vi "loadCal.vi"(8 "error in (no error)":errorcluster, 9 "Wavelength Range (nm)":refnum<vi>, 10 "Center WL (nm)":refnum<vi>, 11 "Type of Measurement":u16(ring)=1 items=["Reflection", "Transmission"]) -> (0 "error out":errorcluster, 2 "valid?":bool)   [LabVIEW 2024]
uses:
  Program Files (x86)/Luna Technologies/OVA 5000 v5.14.2/data/OVA32.dll
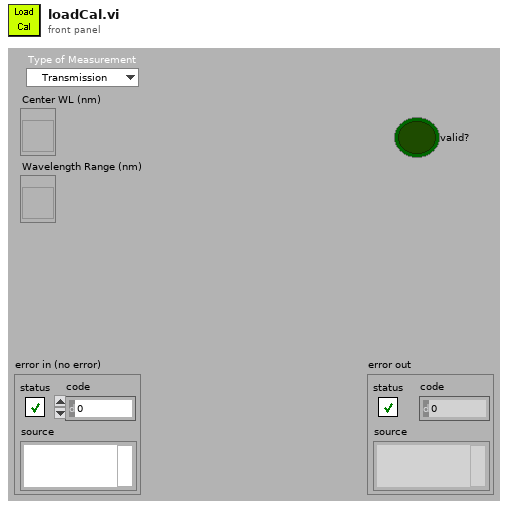
[diagram p1: front panel]
types:
  T1 = cluster{"calStartWL":dbl, "avgs":u32, "timeLength":dbl, "deciFactor":u32, "minStartWL":dbl, "rangeArray":dbl[], "minAvgs":u32, "maxAvgs":u32, "measType":u8, "timeStamp":string, "dutLength":dbl}
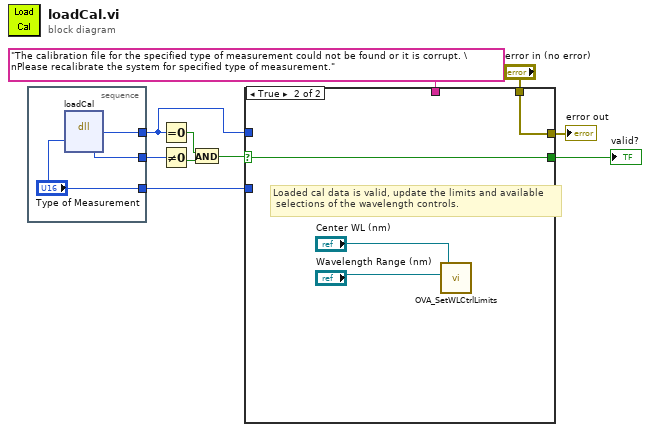
[diagram p0: block diagram]
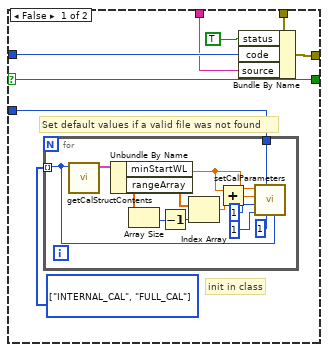
[diagram p2: hidden frame]
diagram:
  n1 = stacked-sequence {
    tunnel: [w13] -> w1
    tunnel: [w12] -> w7
    tunnel: ["Type of Measurement"] -> w6
    frame #0 {
      n2 = dll-call lib="C:/Program Files (x86)/Luna Technologies/OVA 5000 v5.14.2/data/OVA32.dll" fn="loadCal" label="loadCal()"("measType"="Type of Measurement") -> (w13:i32, "valid?"=w12:u8)  [unwired: 5 in, 2 out]
    }
  }
  n3 = Equal To 0?(x=w1) -> (x = 0?=w4:bool)
  n4 = Not Equal To 0?(x=w7) -> (x != 0?=w2:bool)
  n5 = And(x=w4, y=w2) -> (x .and. y?=w3:bool)
  n6 = case shown="True" w3 {
    selector: w3 -> [w14 w34]
    tunnel: "error in (no error)" -> [w21 w37]
    tunnel: [w20 w37] -> w8
    tunnel: w1 -> [w19 _]
    tunnel: "The calibration file for the specified type of measurement could not be found or it is corrupt. \nPlease recalibrate the system for specified type of measurement." -> [w17 _]
    tunnel: w6 -> [w16 _]
    tunnel: [w14 w34] -> w5
    frame False {
      w15 = enum16{"INTERNAL_CAL", "FULL_CAL"}[] [enum."INTERNAL_CAL", enum."FULL_CAL"] items=["INTERNAL_CAL", "FULL_CAL"] ("Array Constant")
      # "init in class"
      # "Set default values if a valid file was not found"
      n7 = for {
        tunnel: w16 -> [w27]
        tunnel: w15 -> [w22] mode=indexing
        n8 = call "getCalStructContents.vi"("calType"=w22) -> ("Calibration Information"=w33:T1)  [unwired: 7 in, 3 out]
        n9 = Unbundle By Name(w33) -> ("minStartWL"=w26:dbl, "rangeArray"=w31:dbl[])
        n10 = Array Size(array=w31) -> (size(s)=w29:i32)
        n11 = Decrement(x=w29) -> (x-1=w30:i32)
        n12 = Index Array(array=w31, index=w30) -> (element=w25:dbl)
        n13 = Add(x=w26, y=w25) -> (x+y=w23:dbl)
        n14 = call "setCalParameters.vi"("calType"=w22, "pdlCal?"=u8 1 ("fullCal?"), "measType"=w27, "deciFactor"=u32 1, "numAvgs"=u32 1, "endWL"=w23, "startWL"=w26) -> ()  [unwired: 5 in]
      }
      n15 = Bundle By Name(cluster=w21, "status"=TRUE, "code"=w19, "source"=w17) -> (w20:errorcluster)
    }
    frame True {
      # "Loaded cal data is valid, update the limits and available\n selections of the wavelength controls."
      n16 = call "OVA_SetWLCtrlLimits.vi"("Wavelength Range (nm)"="Wavelength Range (nm)", "Center WL (nm)"="Center WL (nm)") -> ()  [unwired: 5 in]
    }
  }
  "valid?" <- w5
  "error out" <- w8
